vi "Watchdog Monitor.vi"() -> ()   [LabVIEW 2021]
doc: "This VI continually pings the FPGA watchdog to make sure the time to reset stays high. The real watchdog is in the FPGA. If the timer there isn't continually pinged, the software will reset."
uses:
  <vilib>/Platform/TimedLoop/XDataNode/timing_clust.ctl
  <vilib>/Platform/TimedLoop/XDataNode/nitl_modes.ctl
  <vilib>/Platform/TimedLoop/XDataNode/wakeup.ctl
  <vilib>/Utility/error.llb/Error Cluster From Error Code.vi
  <vilib>/rvi/errors/niLvFpgaAdjustHostInterfaceError.vi
  <vilib>/platform/TimedLoop/XDataNode/XDataNode.xnode
  <vilib>/rvi/interface/nirviReadWriteControl/nirviReadWriteControl.xnode
  <vilib>/Platform/TimedLoop/XDataNode/XDNodeRunTimeDep.lvlib
  NiFpgaLv.dll
  <vilib>/rvi/interface/Simulation/niFpgaSimulationCallBeginRW.vi
panel:
  out "ms Since Whack":u32
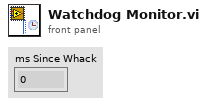
[diagram p1: front panel]
types:
  T1 = typedef "System Resources.ctl" = cluster{"System Session":refnum<k21>, "System Resource":refnum<k20>, "FPGA VI Reference":refnum<k20>}
  T2 = typedef "XDNodeRunTimeDep.lvlib/timing_clust.ctl" = cluster{"Expected End [f-1]":u64, "Actual End [f-1]":u64, "Finished Late? [f-1]":bool, "Expected End [i-1]":u64, "Actual End [i-1]":u64, "Finished Late? [i-1]":bool, "Expected Start [i]":u64, "Actual Start [i]":u64, "Expected Start [f]":u64, "Actual Start [f]":u64, "Source Name":string, "Structure Name":string, "Period":i64, "Deadline":i64, "Offset":i64, "Start":i64, "Priority":i32, "Timeout":i32, "Mode":T3, "Wakeup Reason":T4, "Error":errorcluster, "Source Type":string, "Secondary Source Type":string, "Global End Time":u64, "Global Start Time":u64, "Frame Duration":u64, "Iteration Duration":u64, "Assigned CPU":i32, "I/O Scan Engine Mode":u32}
  T3 = typedef "XDNodeRunTimeDep.lvlib/nitl_modes.ctl" = enum32{"No Change", "Process missed periods, maintain original phase", "Discard missed periods, maintain original phase", "Process missed periods, ignore original phase", "Discard missed periods, ignore original phase"}
  T4 = typedef "XDNodeRunTimeDep.lvlib/wakeup.ctl" = enum32{"Normal", "Aborted", "Asynchronous wakeup", "Timing source error", "Timed loop error", "Timeout"}
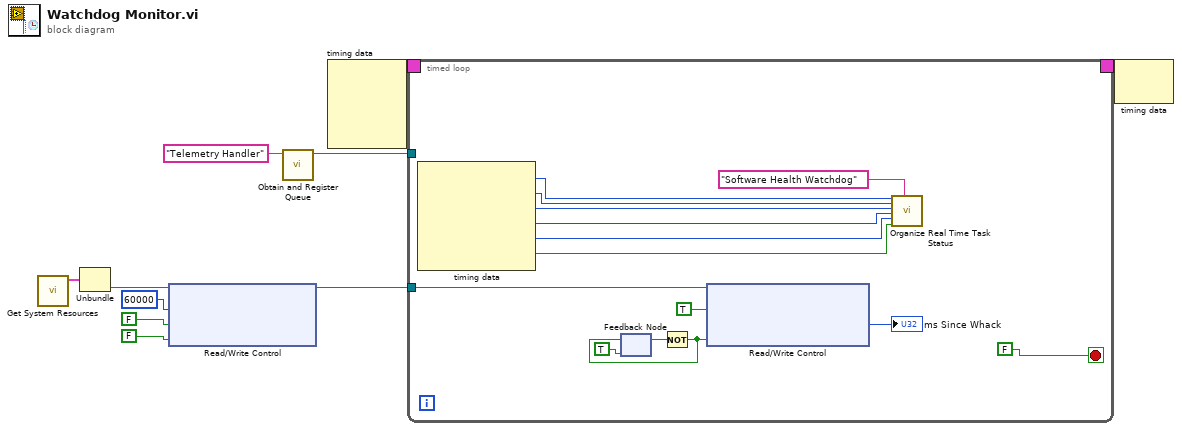
[diagram p0: block diagram]
diagram:
  n1 = call "Get System Resources.vi"() -> ("System Resources"=w5:T1)  [unwired: 10 in, 1 out]
  n2 = Unbundle(w5) -> ("FPGA VI Reference"=w6:refnum<k20>)  [unwired: 2 out]
  n3 = xnode "Read/Write Control"("FPGA VI Reference In"=w6, "Watchdog Timeout (ms)"=u32 60000, "Watchdog Enable"=FALSE ("Enable Watchdog"), "System Reset"=FALSE) -> ("FPGA VI Reference Out"=w7:refnum<k20>)  [unwired: 1 in, 1 out]
  n4 = call "Obtain and Register Queue.vi"("Queue Name (unnamed)"="Telemetry Handler" ("name (unnamed)")) -> ("Queue Reference"=w2:refnum<queue>)  [unwired: 9 in, 1 out]
  n5 = node-c288() -> (w10:T2)  [unwired: 4 in]
  n6 = timed-loop {
    timing: w10 -> [_]
    timing-out: [_] -> w9
    tunnel: w2 -> [_]
    tunnel: w7 -> [w15]
    stop <- FALSE stop-if-true
    n7 = node-c288() -> (w22:i32, w21:i32, w20:i64, w19:i64, w18:i64, w17:bool)  [unwired: 1 in]
    n8 = feedback #1(TRUE ("Whack")) -> (w12:bool)
    n9 = Not(x=w12) -> (.not. x?=w11:bool)
    n10 = feedback-in #1(w11) -> ()
    n11 = xnode "Read/Write Control"("FPGA VI Reference In"=w15, "Watchdog Whack"=TRUE ("Whack"), "FPGA USER1 LED"=w11) -> ("Watchdog ms Since Whack"=→"ms Since Whack":u32)  [unwired: 1 in, 2 out]
    n12 = call "Organize Real Time Task Status.vi"("Priority"=w22, "Processor"=w21, "Offset"=w20, "Iteration Duration"=w19, "Period"=w18, "Finished Late? [i-1]"=w17, "Task Name"="Software Health Watchdog") -> ()  [unwired: 12 in, 1 out]
  }
  n13 = node-c288(w9) -> ()  [unwired: 1 out]
